vi "Change from tunnel to model coordinates.vi"() -> (0 "error out":errorcluster, 4 "Path":path)   [LabVIEW 2014]
panel:
  out "File Changed":bool
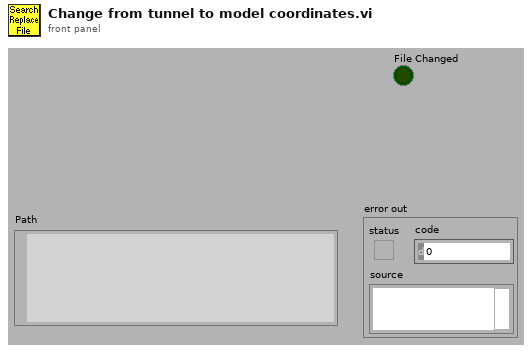
[diagram p1: front panel]
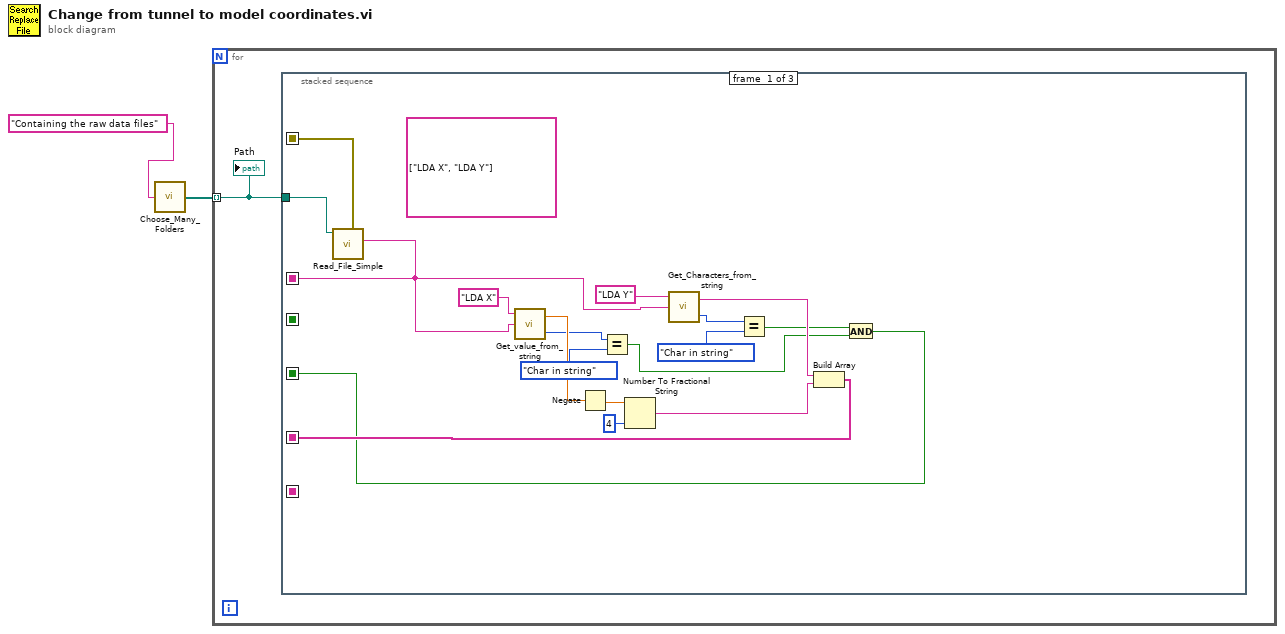
[diagram p0: block diagram]
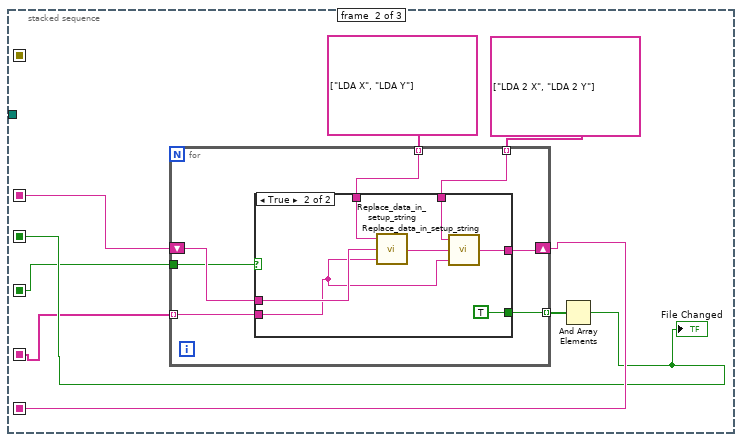
[diagram p2: hidden frame]
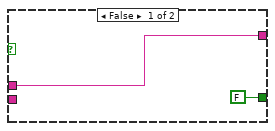
[diagram p3: hidden frame]
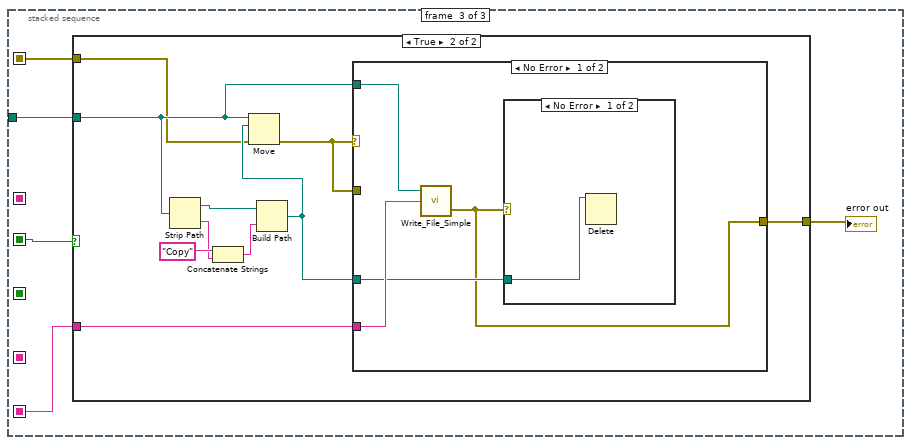
[diagram p4: hidden frame]
diagram:
  n1 = call "Choose_Many_Folders.vi"("Purpose of choosing folder"="Containing the raw data files") -> ("Files"=w1:path[])
  n2 = for {
    tunnel: w1 -> [w3] mode=indexing
    n3 = stacked-sequence {
      seq-local: [w20 _ _] -> [_ _ w46]
      seq-local: [_ w28 _] -> [_ _ w48]
      seq-local: [_ w25 _] -> [_ _ w47]
      seq-local: [w14 _ _] -> [_ w24 _]
      seq-local: [w11 _ _] -> [_ w22 _]
      seq-local: [w4 _ _] -> [_ w23 _]
      tunnel: w3 -> [w21 _ w50]
      frame #0 {
        (unwired) string[] ["LDA X", "LDA Y"]
        n4 = call "Read_File_Simple.vi"("Filename"=w21) -> ("error out"=w20:errorcluster, "string"=w14:string)  [unwired: 4 in, 4 out]
        n5 = call "Get_value_from_string.vi"("Input string"=w14, "Variable name"="LDA X" ("Output String")) -> ("Status"=w8:enum16{"Char in string", "Char not in string"}, "Value"=w18:dbl)  [unwired: 1 in]
        n6 = Negate(x=w18) -> (-x=w17:dbl)
        n7 = Equal?(x=w8, y=enum16{"Char in string", "Char not in string"}."Char in string" ("Status")) -> (x = y?=w5:bool)
        n8 = Number To Fractional String(number=w17, precision (6)=i16 4) -> (F-format string=w12:string)  [unwired: 2 in]
        n9 = call "Get_Characters_from_string.vi"("Input string"=w14, "Variable name"="LDA Y" ("Output String")) -> ("Status"=w9:enum16{"Char in string", "Char not in string"}, "Value"=w13:string)  [unwired: 1 in]
        n10 = Equal?(x=w9, y=enum16{"Char in string", "Char not in string"}."Char in string" ("Status")) -> (x = y?=w6:bool)
        n11 = Build Array(w13, w12) -> (w11:string[])
        n12 = And(x=w6, y=w5) -> (x .and. y?=w4:bool)
      }
      frame #1 {
        n13 = for {
          shift-right: [w33] -> w28
          shift-left: w24 -> [w34]
          tunnel: string[] ["LDA X", "LDA Y"] -> [w36] mode=indexing
          tunnel: string[] ["LDA 2 X", "LDA 2 Y"] -> [w35] mode=indexing
          tunnel: [w32] -> w26 mode=indexing
          tunnel: w23 -> [w31]
          tunnel: w22 -> [w30] mode=indexing
          n14 = case shown="True" w31 {
            tunnel: w36 -> [_ w45]
            tunnel: w35 -> [_ w44]
            tunnel: w34 -> [w38 w43]
            tunnel: [w38 w42] -> w33
            tunnel: [FALSE TRUE] -> w32
            tunnel: w30 -> [_ w39]
            frame False {
            }
            frame True {
              n15 = call "Replace_data_in_setup_string.vi"("New data string"=w39, "Input string"=w43, "Variable name"=w45) -> ("Appended string"=w41:string)
              n16 = call "Replace_data_in_setup_string.vi"("New data string"=w39, "Input string"=w41, "Variable name"=w44) -> ("Appended string"=w42:string)
            }
          }
        }
        n17 = And Array Elements(Boolean array=w26) -> (logical AND=w25:bool)
        "File Changed" <- w25
      }
      frame #2 {
        n18 = case shown="True" w47 {
          tunnel: w50 -> [_ w57]
          tunnel: w48 -> [_ w56]
          tunnel: [w51 w54] -> w49
          tunnel: w46 -> [w51 w52]
          frame False {
          }
          frame True {
            n19 = Strip Path(path=w57) -> (stripped path=w58:path, name=w60:string)
            n20 = Concatenate Strings("Copy" ("name or relative path"), w60) -> (w59:string)
            n21 = Build Path(base path=w58, name or relative path=w59) -> (appended path=w55:path)
            n22 = Move(source path=w57, error in=w52, 10:w55) -> (error out=w53:errorcluster)  [unwired: 2 in, 2 out]
            n23 = case shown="No Error" w53 {
              tunnel: w57 -> [w65 _]
              tunnel: w56 -> [w64 _]
              tunnel: w55 -> [w63 _]
              tunnel: [w62 w67] -> w54
              tunnel: w53 -> [_ w67]
              frame No Error {
                n24 = call "Write_File_Simple.vi"("character string"=w64, "file path"=w65) -> ("error out"=w62:errorcluster)  [unwired: 1 in, 1 out]
                n25 = case shown="No Error" w62 {
                  tunnel: w63 -> [w66 _]
                  frame No Error {
                    n26 = Delete(path (use dialog)=w66) -> ()  [unwired: 4 in, 3 out]
                  }
                  frame Error {
                  }
                }
              }
              frame Error {
              }
            }
          }
        }
        "error out" <- w49
      }
    }
    "Path" <- w3
  }
